vi "Take.vi"(11 "dy":dbl) -> ()   [LabVIEW 2015]
uses:
  Global Distance.vi
  Global Angle.vi
panel:
  out "x*y":dbl
  in  "dz input":dbl(slide) scale=0.0..130.0
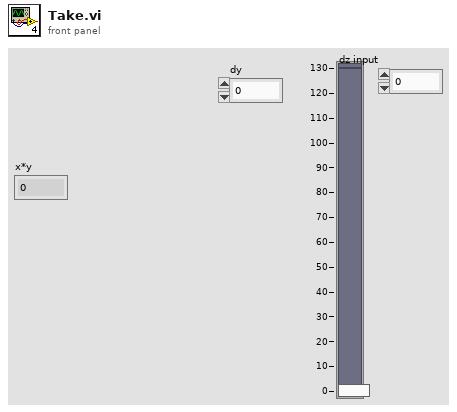
[diagram p1: front panel]
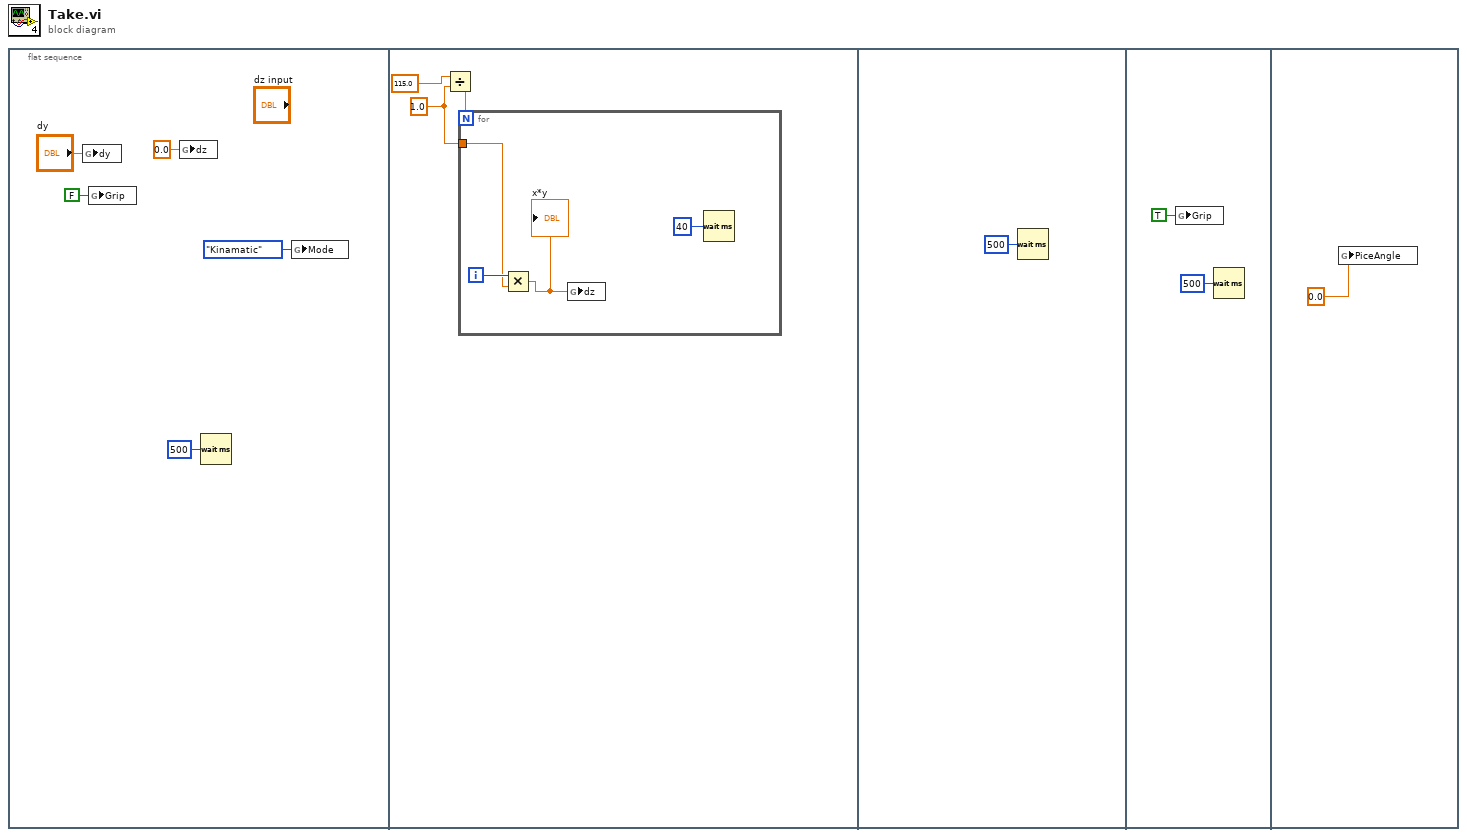
[diagram p0: block diagram]
diagram:
  n1 = flat-sequence {
    frame #0 {
      n2 = global write "Global Distance.vi" "dy"("dy") -> ()
      n3 = global write "Global Angle.vi" "Grip"(FALSE ("Grip")) -> ()
      n4 = global write "Global Distance.vi" "dz"(0.0 ("dz")) -> ()
      n5 = Wait (ms)(milliseconds to wait=u32 500) -> ()  [unwired: 1 out]
      n6 = global write "Global Angle.vi" "Mode"(enum16{"Normal", "Zero", "Kinamatic", "Camera"}."Kinamatic" ("Mode")) -> ()
    }
    frame #1 {
      w6 = 1.0 ("y")
      n7 = Divide(x=115.0 ("z limit"), y=w6) -> (x/y=w8:dbl)
      n8 = for {
        N: w8 -> [_]
        tunnel: w6 -> [w9]
        i -> [w11]
        n9 = Multiply(x=w11, y=w9) -> (x*y=w10:dbl)
        "x*y" <- w10
        n10 = global write "Global Distance.vi" "dz"(w10) -> ()
        n11 = Wait (ms)(milliseconds to wait=u32 40) -> ()  [unwired: 1 out]
      }
    }
    frame #2 {
      n12 = Wait (ms)(milliseconds to wait=u32 500) -> ()  [unwired: 1 out]
    }
    frame #3 {
      n13 = global write "Global Angle.vi" "Grip"(TRUE ("Grip")) -> ()
      n14 = Wait (ms)(milliseconds to wait=u32 500) -> ()  [unwired: 1 out]
    }
    frame #4 {
      n15 = global write "Global Angle.vi" "PiceAngle"(0.0 ("PiceAngle")) -> ()
    }
  }
